vi "VelocityController.vi"(8 "error in (no error)":errorcluster) -> (0 "error out":errorcluster)   [LabVIEW 2013]
uses:
  My Computer/Controls/Steering Inputs.ctl
  My Computer/Controls/SpaceMouse_FilteredInput.ctl
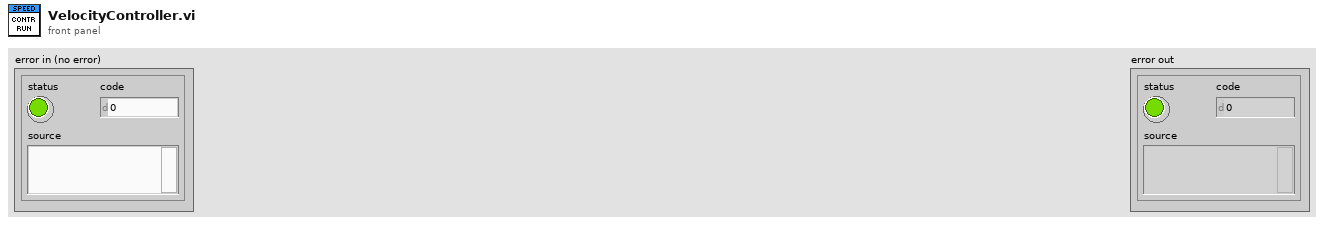
[diagram p1: front panel]
types:
  T1 = typedef "Steering Inputs.ctl" = cluster{"X":dbl, "Y":dbl, "Z":dbl, "phi":dbl, "theta":dbl, "psi":dbl}
  T2 = cluster{"u_B_des":dbl, "v_B_des":dbl, "w_B_des":dbl}
  T3 = typedef "SpaceMouse_FilteredInput.ctl" = cluster{"X":dbl, "Y":dbl, "Z":dbl, "phi":dbl, "theta":dbl, "psi":dbl}
  T4 = cluster{"ARW on":cluster{"u":bool, "v":bool, "w":bool}, "kp":cluster{"kp_u":dbl, "kp_v":dbl, "kp_w":dbl}, "Ti":cluster{"Ti_u":dbl, "Ti_v":dbl, "Ti_w":dbl}, "Integrator enabled range [rad      ":cluster{"I_E_u":dbl, "I_E_v":dbl, "I_E_w":dbl}}
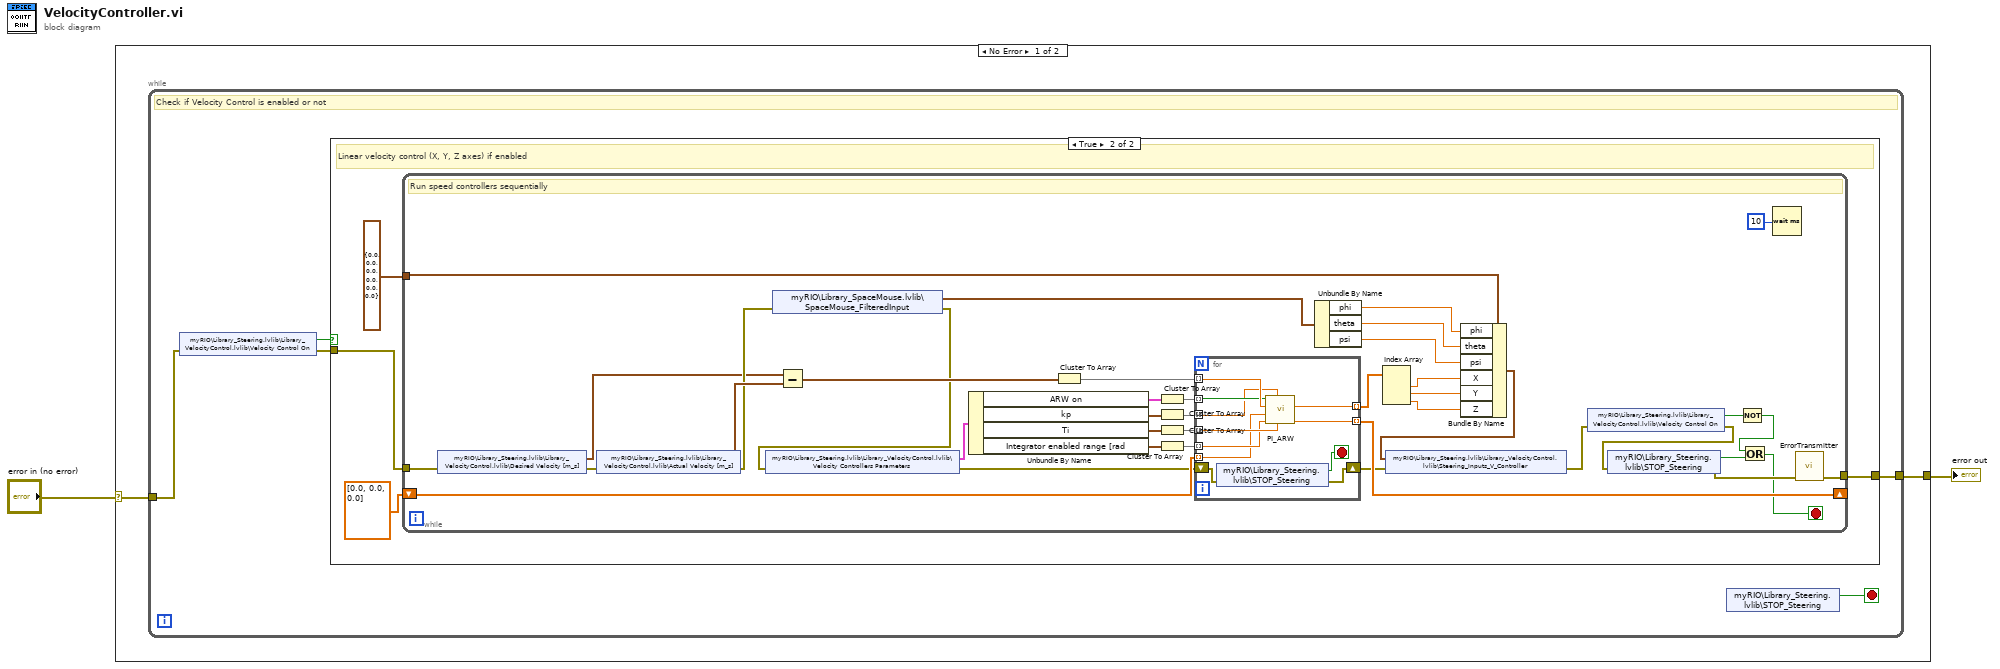
[diagram p0: block diagram]
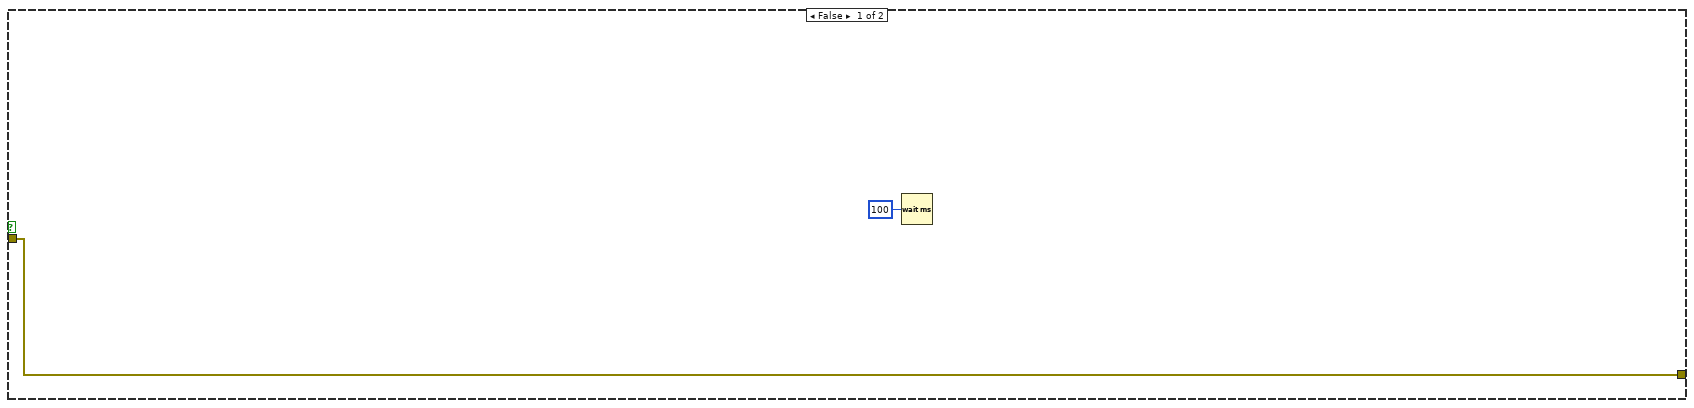
[diagram p2: hidden frame]
diagram:
  n1 = case shown="No Error" "error in (no error)" {
    selector: "error in (no error)" -> [w3 w67]
    tunnel: [w4 w67] -> w2
    frame No Error {
      n2 = while {
        tunnel: w3 -> [w6]
        tunnel: [w9] -> w4
        stop <- w7 stop-if-true
        # "Check if Velocity Control is enabled or not"
        n3 = shared-variable "myRIO\\Library_Steering.lvlib\\Library_VelocityControl.lvlib\\Velocity Control On"(error in=w6) -> (w8:bool, error out=w5:errorcluster)
        n4 = case shown="True" w8 {
          tunnel: [w10 w12] -> w9
          tunnel: w5 -> [w10 w13]
          frame False {
            n5 = Wait (ms)(milliseconds to wait=u32 100) -> ()  [unwired: 1 out]
          }
          frame True {
            # "Linear velocity control (X, Y, Z axes) if enabled"
            n6 = while {
              shift-right: [w44] -> _
              shift-left: dbl[] [0.0, 0.0, 0.0] -> [w43]
              tunnel: w13 -> [w25]
              tunnel: [w40] -> w12
              tunnel: T1 {"X"=0.0, "Y"=0.0, "Z"=0.0, "phi"=0.0, "theta"=0.0, "psi"=0.0} ("Steering_Inputs_A_Controller") -> [w38]
              stop <- w32 stop-if-true
              # "Run speed controllers sequentially"
              n7 = shared-variable "myRIO\\Library_Steering.lvlib\\Library_VelocityControl.lvlib\\Desired Velocity [m_s]"(error in=w25) -> (w26:T2, error out=w24:errorcluster)
              n8 = shared-variable "myRIO\\Library_Steering.lvlib\\Library_VelocityControl.lvlib\\Actual Velocity [m_s]"(error in=w24) -> (w55:cluster{"u_B":dbl, "v_B":dbl, "w_B":dbl}, error out=w27:errorcluster)
              n9 = shared-variable "myRIO\\Library_SpaceMouse.lvlib\\SpaceMouse_FilteredInput"(error in=w27) -> (w31:T3, error out=w19:errorcluster)
              n10 = shared-variable "myRIO\\Library_Steering.lvlib\\Library_VelocityControl.lvlib\\Velocity Controllers Parameters"(error in=w19) -> (w21:T4, error out=w20:errorcluster)
              n11 = Subtract(x=w26, y=w55) -> (x-y=w54:cluster{dbl, dbl, dbl})
              n12 = Unbundle By Name(w21) -> ("ARW on"=w52:cluster{"u":bool, "v":bool, "w":bool}, "kp"=w49:cluster{"kp_u":dbl, "kp_v":dbl, "kp_w":dbl}, "Ti"=w50:cluster{"Ti_u":dbl, "Ti_v":dbl, "Ti_w":dbl}, "Integrator enabled range [rad"=w51:cluster{"I_E_u":dbl, "I_E_v":dbl, "I_E_w":dbl})
              n13 = Cluster To Array(cluster=w54) -> (array=w53:dbl[])
              n14 = Cluster To Array(cluster=w52) -> (array=w48:bool[])
              n15 = Cluster To Array(cluster=w49) -> (array=w47:dbl[])
              n16 = Cluster To Array(cluster=w50) -> (array=w46:dbl[])
              n17 = Cluster To Array(cluster=w51) -> (array=w45:dbl[])
              n18 = for {
                tunnel: w53 -> [w66] mode=indexing
                tunnel: w48 -> [w65] mode=indexing
                tunnel: w47 -> [w64] mode=indexing
                tunnel: w46 -> [w63] mode=indexing
                tunnel: w45 -> [w62] mode=indexing
                tunnel: [w61] -> w39 mode=indexing
                tunnel: [w60] -> w44 mode=indexing
                tunnel: w43 -> [w59] mode=indexing
                shift-right: [w56] -> w17
                shift-left: w20 -> [w57]
                stop <- w58 stop-if-true
                n19 = shared-variable "myRIO\\Library_Steering.lvlib\\STOP_Steering"(error in=w57) -> (w58:bool, error out=w56:errorcluster)
                n20 = call "PI_ARW.vi"("Ti_value"=w63, "p_value"=w64, "Integrator enabled range"=w62, "old error"=w59, "actual error"=w66, "ARW on/off"=w65) -> ("new error"=w60:dbl, "output"=w61:dbl)  [unwired: 2 in]
              }
              n21 = Unbundle By Name(w31) -> ("phi"=w30:dbl, "theta"=w29:dbl, "psi"=w28:dbl)
              n22 = Index Array(array=w39) -> (element #1=w22:dbl, element #2=w37:dbl, element #3=w23:dbl)  [unwired: 3 in]
              n23 = Bundle By Name(cluster=w38, "phi"=w30, "theta"=w29, "psi"=w28, "X"=w22, "Y"=w37, "Z"=w23) -> (w16:T1)
              n24 = shared-variable "myRIO\\Library_Steering.lvlib\\Library_VelocityControl.lvlib\\Steering_Inputs_V_Controller"(w16, error in=w17) -> (error out=w18:errorcluster)
              n25 = shared-variable "myRIO\\Library_Steering.lvlib\\Library_VelocityControl.lvlib\\Velocity Control On"(error in=w18) -> (w36:bool, error out=w35:errorcluster)
              n26 = shared-variable "myRIO\\Library_Steering.lvlib\\STOP_Steering"(error in=w35) -> (w34:bool, error out=w41:errorcluster)
              n27 = Not(x=w36) -> (.not. x?=w33:bool)
              n28 = Or(x=w33, y=w34) -> (x .or. y?=w32:bool)
              n29 = Wait (ms)(milliseconds to wait=u32 10) -> ()  [unwired: 1 out]
              n30 = call "ErrorTransmitter.vi"("Error In"=w41) -> ("Error Out"=w40:errorcluster)  [unwired: 10 in]
            }
          }
        }
        n31 = shared-variable "myRIO\\Library_Steering.lvlib\\STOP_Steering"() -> (w7:bool)  [unwired: 1 in, 1 out]
      }
    }
    frame Error {
    }
  }
  "error out" <- w2
